vi "gfitsio-create-img.vi"(4 "image data type":T1 items=["<invalid type>"=0, "BYTE_IMG  (U8)"=8, "SHORT_IMG  (I16)"=16, "USHORT_IMG  (U16)"=20, "LONG_IMG  (I32)"=32, "ULONG_IMG  (U32)"=40, "FLOAT_IMG  (SGL)"=-32, "DOUBLE_IMG  (DBL)"=-64], 6 "naxes":i32[](array[numeric]), 7 "extname":string, 8 "error in (no error)":errorcluster, 11 "gfits refnum":T2) -> (0 "error out":errorcluster, 3 "dup gfits refnum":T2)   [LabVIEW 2019, in "gfitsio.lvlib"]
doc: "Create a new IMAGE extension with a specified data type and size."
uses:
  gfitsio.lvlib
  gfitsio-refnum.ctl
  cfitsio-bitpix.ctl
  gfitsio-error-codes.ctl
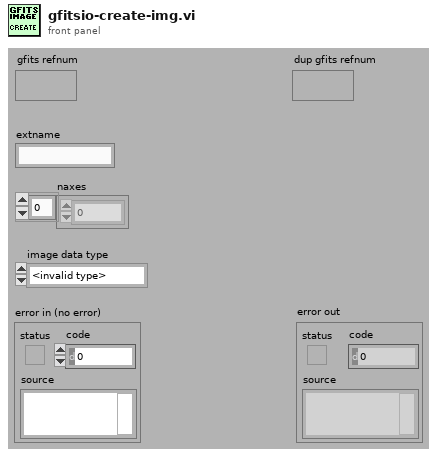
[diagram p1: front panel]
types:
  T1 = typedef "gfitsio.lvlib/cfitsio-bitpix.ctl" = i32
  T2 = typedef "gfitsio.lvlib/gfitsio-refnum.ctl" = refnum<k1>
  T3 = typedef "gfitsio.lvlib/gfitsio-error-codes.ctl" = i32
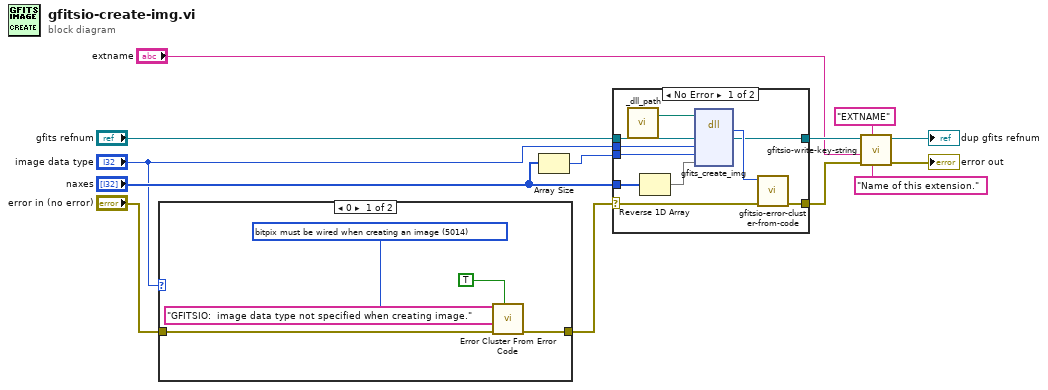
[diagram p0: block diagram]
diagram:
  n1 = case shown="0" "image data type" {
    tunnel: "error in (no error)" -> [w17 w19]
    tunnel: [w18 w19] -> w2
    frame 0 {
      w16 = T3 5014 items=["no error"=0, "dimensionality conflict"=5001, "fpixel out of image bounds"=5002, "lpixel out of image bounds"=5003, "increment size larger than image"=5004, "increment must be greater than zero"=5005, "fpixel must specify lower left corner"=5006, "named HDU not found"=5007, "specified row is past the end of the table"=5008, "wrong number of elements for column"=5009, "column is not scalar"=5010, "duplicate HDU name"=5011, "invalid table type"=5012, "row counting starts at 1"=5013, "bitpix must be wired when creating an image"=5014] ("Ring")
      n2 = call <vilib>:"Error Cluster From Error Code.vi"("show call chain? (False)"=TRUE, "error in (no error)"=w17, "error message (\"\")"="GFITSIO:  image data type not specified when creating image." ("error message (\"\")"), "error code (0)"=w16) -> ("error out"=w18:errorcluster)  [unwired: 5 out]
    }
    frame Default {
    }
  }
  n3 = Array Size(array="naxes") -> (size(s)=w11:i32)
  n4 = case shown="No Error" w2 {
    selector: w2 -> [w27 w31]
    tunnel: [w29 w31] -> w8
    tunnel: "naxes" -> [w23 _]
    tunnel: "gfits refnum" -> [w25 w30]
    tunnel: [w26 w30] -> w7
    tunnel: w11 -> [w24 _]
    tunnel: "image data type" -> [w22 _]
    frame No Error {
      n5 = call "_dll_path.vi"() -> ("Path"=w20:path)  [unwired: 1 in]
      n6 = Reverse 1D Array(array=w23) -> (reversed array=w21:i32[])
      n7 = dll-call lib="?" fn="gfits_create_img"(path in=w20, "refnum"=w25, "bitpix"=w22, "naxis"=w24, "naxes"=w21) -> ("return type"=w28:i32, "refnum"=w26:T2)  [unwired: 4 in, 3 out]
      n8 = call "gfitsio-error-cluster-from-code.vi"("error in (no error)"=w27, "error code"=w28) -> ("error out"=w29:errorcluster)  [unwired: 9 out]
    }
    frame Error {
    }
  }
  n9 = call "gfitsio-write-key-string.vi"("comment"="Name of this extension.", "keyname"="EXTNAME", "error in (no error)"=w8, "value"="extname", "gfits refnum"=w7) -> ("error out"=→"error out":errorcluster, "dup gfits refnum"=→"dup gfits refnum":T2)  [unwired: 5 out]
